vi "Clicked.vi"(8 "error in (no error)":errorcluster, 9 "Siblings":refnum<data-value>[](array[refnum]), 10 "Clicked Tag":string, 11 "MGI_MenuItem in":refnum<class "MGI_MenuItem.lvclass">) -> (0 "error out":errorcluster, 3 "MGI_MenuItem out":refnum<class "MGI_MenuItem.lvclass">)   [LabVIEW 2016, in "MGI_MenuItem.lvclass"]
doc: "This VI is called when a menu is clicked. It recursively searchs its self and it's sub menus to see if it is the menu item that has been clicked.\n\nAuthored by Derek E. Trepanier\nsupport@mooregoodideas.com\nwww.mooregoodideas.com\n\nCopyright (c) 2012, Moore Good Ideas, Inc.\n\nAll rights reserved.\n\nRedistribution and use in source and binary forms, with or without modification, are permitted provided that the following conditions are met:\n\n * Redistributions of source code must retain the above copyright notice, this list of conditions and the following disclaimer.\n * Redistributions in binary form must reproduce the above copyright notice, this list of conditions and the following disclaimer in the documentation and/or other materials provided with the distribution.\n * Neither the name of Moore Good Ideas, Inc. nor the names of its contributors may be used to endorse or promote products derived from this software without specific prior written permission.\n\nTHIS SOFTWARE IS PROVIDED BY THE COPYRIGHT HOLDERS AND CONTRIBUTORS \"AS IS\" AND ANY EXPRESS OR IMPLIED WARRANTIES, INCLUDING, BUT NOT LIMITED TO, THE IMPLIED WARRANTIES OF MERCHANTABILITY AND FITNESS FOR A PARTICULAR PURPOSE ARE DISCLAIMED. IN NO EVENT SHALL THE COPYRIGHT OWNER OR CONTRIBUTORS BE LIABLE FOR ANY DIRECT, INDIRECT, INCIDENTAL, SPECIAL, EXEMPLARY, OR CONSEQUENTIAL DAMAGES (INCLUDING, BUT NOT LIMITED TO, PROCUREMENT OF SUBSTITUTE GOODS OR SERVICES; LOSS OF USE, DATA, OR PROFITS; OR BUSINESS INTERRUPTION) HOWEVER CAUSED AND ON ANY THEORY OF LIABILITY, WHETHER IN CONTRACT, STRICT LIABILITY, OR TORT (INCLUDING NEGLIGENCE OR OTHERWISE) ARISING IN ANY WAY OUT OF THE USE OF THIS SOFTWARE, EVEN IF ADVISED OF THE POSSIBILITY OF SUCH DAMAGE."
uses:
  <userlib>/_MGI/Menu Building/MenuItem/MGI_MenuItem.lvclass
  <userlib>/_MGI/Menu Building/MenuItem/Read Sub-Menus.vi
  <userlib>/_MGI/Menu Building/MenuItem/Read Tag.vi
  <userlib>/_MGI/Menu Building/MenuItem/Read SelectionType.vi
  <userlib>/_MGI/Menu Building/SelectionType/MGI_SelectionType.lvclass
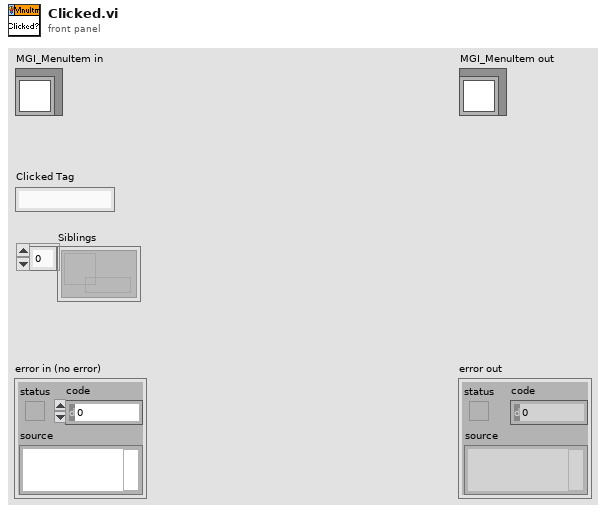
[diagram p1: front panel]
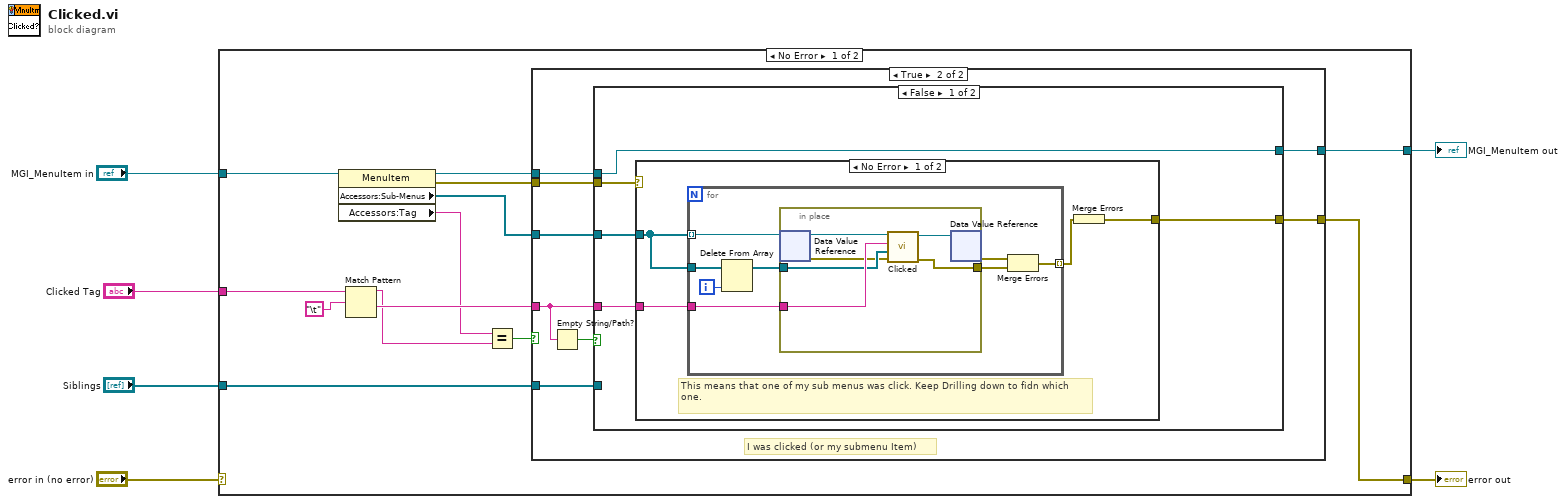
[diagram p0: block diagram]
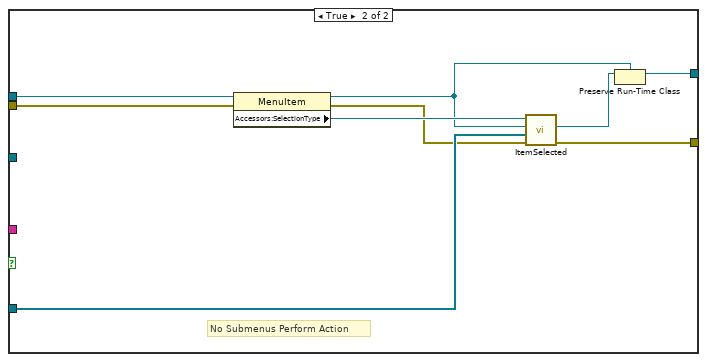
[diagram p4: hidden frame]
diagram:
  n1 = case shown="No Error" "error in (no error)" {
    selector: "error in (no error)" -> [_ w64]
    tunnel: [w9 w64] -> w5
    tunnel: [w14 w63] -> w3
    tunnel: "MGI_MenuItem in" -> [w18 w63]
    tunnel: "Clicked Tag" -> [w8 _]
    tunnel: "Siblings" -> [w16 _]
    frame No Error {
      n2 = property class="MenuItem"(reference=w18) -> (reference out=w15:refnum<class "MGI_MenuItem.lvclass">, error out=w10:errorcluster, "Accessors:Sub-Menus"=w17:refnum<data-value>[], "Accessors:Tag"=w12:string)  [unwired: 1 in]
      n3 = Match Pattern(string=w8, regular expression="\t") -> (before substring=w11:string, after substring=w13:string)  [unwired: 1 in, 2 out]
      n4 = Equal?(x=w12, y=w11) -> (x = y?=w19:bool)
      n5 = case shown="True" w19 {
        tunnel: w13 -> [_ w24]
        tunnel: w17 -> [_ w29]
        tunnel: w16 -> [_ w28]
        tunnel: w15 -> [w21 w27]
        tunnel: [w21 w26] -> w14
        tunnel: w10 -> [w20 w23]
        tunnel: [w20 w22] -> w9
        frame False {
          # "Not part of the clicked chain. Do nothing"
        }
        frame True {
          # "I was clicked (or my submenu Item)"
          n6 = Empty String/Path?(string/path=w24) -> (empty?=w25:bool)
          n7 = case shown="False" w25 {
            tunnel: w24 -> [w31 _]
            tunnel: w29 -> [w32 _]
            tunnel: w28 -> [_ w61]
            tunnel: w27 -> [w34 w58]
            tunnel: [w34 w56] -> w26
            tunnel: w23 -> [w30 w57]
            tunnel: [w33 w59] -> w22
            frame False {
              n8 = case shown="No Error" w30 {
                selector: w30 -> [_ w53]
                tunnel: [w38 w53] -> w33
                tunnel: w32 -> [w37 _]
                tunnel: w31 -> [w36 _]
                frame No Error {
                  # "This means that one of my sub menus was click. Keep Drilling down to fidn which one."
                  n9 = for {
                    tunnel: w37 -> [w44] mode=indexing
                    tunnel: w36 -> [w46]
                    tunnel: w37 -> [w45]
                    tunnel: [w41] -> w35 mode=indexing
                    i -> [w39]
                    n10 = Delete From Array(array=w45, index=w39) -> (array with subset deleted=w40:refnum<data-value>[])  [unwired: 1 in, 1 out]
                    n11 = in-place {
                      in-place-border: w46 -> [w52]
                      in-place-border: w40 -> [w48]
                      in-place-border: [w50] -> w42
                      n12 = in-place-dvr #1(w44) -> (w49:refnum<class "MGI_MenuItem.lvclass">, w47:errorcluster)
                      n13 = call-dynamic "Clicked.vi"("error in (no error)"=w47, "Siblings"=w48, "Clicked Tag"=w52, "MGI_MenuItem in"=w49) -> ("error out"=w50:errorcluster, "MGI_MenuItem out"=w51:refnum<class "MGI_MenuItem.lvclass">)  [unwired: 6 in]
                      n14 = in-place-dvr #1(w51) -> (w43:errorcluster)  [unwired: 1 out]
                    }
                    n15 = Merge Errors(w43, w42) -> (w41:errorcluster)
                  }
                  n16 = Merge Errors(w35) -> (w38:errorcluster)
                }
                frame Error {
                }
              }
            }
            frame True {
              # "No Submenus Perform Action"
              n17 = property class="MenuItem"(reference=w58, error in=w57) -> (reference out=w55:refnum<class "MGI_MenuItem.lvclass">, error out=w60:errorcluster, "Accessors:SelectionType"=w62:refnum<class "MGI_SelectionType.lvclass">)
              n18 = call-dynamic "ItemSelected.vi"("error in (no error)"=w60, "Siblings"=w61, "MenuItem in"=w55, "SelectionType in"=w62) -> ("error out"=w59:errorcluster, "MenuItem out"=w54:refnum<class "MGI_MenuItem.lvclass">)  [unwired: 5 in, 1 out]
              n19 = Preserve Run-Time Class(object in=w54, 2:w55) -> (object out=w56:refnum<class "MGI_MenuItem.lvclass">)  [unwired: 1 in, 1 out]
            }
          }
        }
      }
    }
    frame Error {
    }
  }
  "error out" <- w5
  "MGI_MenuItem out" <- w3
